vi "HasTransitionFailed.vi"(8 "Robot heading (deg)":dbl format="%#_13g", 9 "Trusted absolute wind (deg)":dbl format="%#_13g", 11 "Last Commanded Sailing Regime":T1) -> (3 "HasTransitionFailed?":bool)   [LabVIEW 2013]
doc: "This VI should check whether the boat has failed the transition it is in, and it should only be called if the boat is currently in a transition state.\n\nAt the moment the thought is that only a tack can fail, jibes and turning without crossing the wind should never be ruled as failed. This is because in a jibe or turn there is always force on the boat to let it keep trying to turn, and in a tack if the boat gets stuck in irons there isn't any useful force on the boat. At that point keeping on trying to turn won't get anywhere, and a 'failed' flag should be raised.\n\nEric Schneider, Feb, 2014"
uses:
  Data/TypeDefs/Sailing Regimes.ctl
  Utilities/Math/Angles/Angle/Angle.lvclass
panel:
  out "Restart timer 1?":bool
  out "index":i32
  out "Timer 2: Time since last reset":dbl
  out "Time since last reset command":dbl
  in  "stop":bool
  out "Reset timer 2?":bool
  in  "Angle to wind considered 'in irons' (deg)":dbl=40.0 format="%#_13g"
  in  "Time elapsed before tack is considered failed (s)":dbl=8.0 format="%#_13g"
  # "SET TO A DEFAULT, TUNE THIS BY HAND\nIF YOU HAVE PROBLEMS WITH IT"
  # "SET TO A DEFAULT, TUNE THIS BY HAND\nIF YOU HAVE PROBLEMS WITH IT"
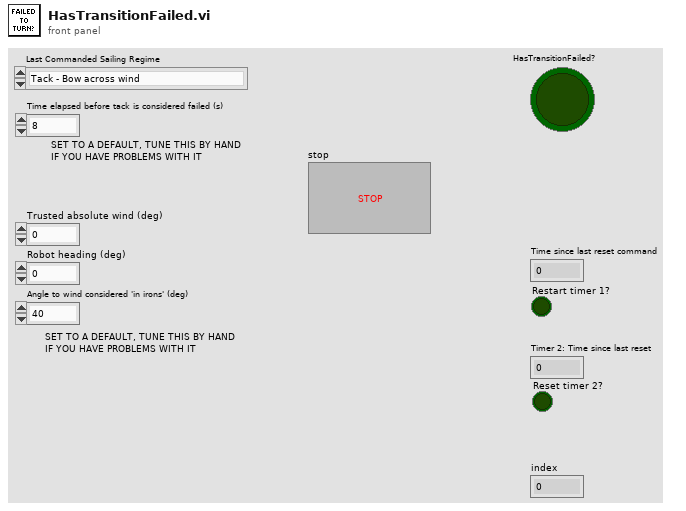
[diagram p1: front panel]
types:
  T1 = typedef "Sailing Regimes.ctl" = enum16{"Tack - Bow across wind", "Upwind - Port Tack", "Turn between Upwind/Reach - Port Tack", "Reach - Port Tack", "Turn between Reach/Run - Port Tack", "Run - Port Tack", "Jibe - Stern across wind", "Run - Starboard Tack", "Turn between Reach/Run - Starboard Tack", "Reach - Starboard Tack", "Turn between Upwind/Reach - Starboard Tack", "Upwind - Starboard Tack"}
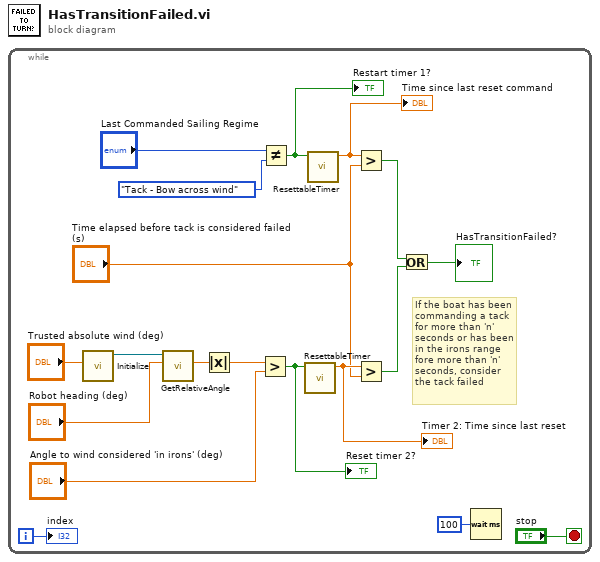
[diagram p0: block diagram]
diagram:
  n1 = while {
    i -> [w2]
    stop <- "stop" stop-if-true
    # "If the boat has been commanding a tack for more than 'n' seconds or has been in the irons range fore more than 'n' seconds, consider the tack failed"
    n2 = call "Initialize.vi"("Input Angle (Deg.)"="Trusted absolute wind (deg)") -> ("Angle out"=w14:refnum<class "Angle.lvclass">)  [unwired: 9 in, 1 out]
    n3 = call "GetRelativeAngle.vi"("Boat Heading (Deg.)"="Robot heading (deg)", "Angle in"=w14) -> ("Relative Angle"=w12:dbl)  [unwired: 8 in, 1 out]
    n4 = Absolute Value(x=w12) -> (abs(x)=w11:dbl)
    n5 = Greater?(x=w11, y="Angle to wind considered 'in irons' (deg)") -> (0:w10:bool)
    "Reset timer 2?" <- w10
    n6 = Not Equal?(x="Last Commanded Sailing Regime", y=Sailing_Regimes."Tack - Bow across wind") -> (x != y?=w17:bool)
    "Restart timer 1?" <- w17
    n7 = call "ResettableTimer.vi"("Restart timer?"=w10) -> ("Time since last reset"=w7:dbl)  [unwired: 10 in]
    "Timer 2: Time since last reset" <- w7
    n8 = call "ResettableTimer.vi"("Restart timer?"=w17) -> ("Time since last reset"=w16:dbl)  [unwired: 10 in]
    "Time since last reset command" <- w16
    n9 = Greater?(x=w16, y="Time elapsed before tack is considered failed (s)") -> (0:w8:bool)
    n10 = Greater?(x=w7, y="Time elapsed before tack is considered failed (s)") -> (0:w5:bool)
    n11 = Or(x=w8, y=w5) -> (x .or. y?=→"HasTransitionFailed?":bool)
    n12 = Wait (ms)(milliseconds to wait=u32 100) -> ()  [unwired: 1 out]
    "index" <- w2
  }
